vi "Read InTemperatureRange.vi"(8 "error in (no error)":errorcluster, 11 "CoolerControler in":refnum<class "CoolerControler.lvclass">) -> (0 "error out":errorcluster, 2 "InTemperatureRange":dbl=3.0, 3 "CoolerControler out":refnum<class "CoolerControler.lvclass">)   [LabVIEW 2016, in "CoolerControler.lvclass"]
uses:
  CoolerControler.lvclass
  CoolerControler.lvclass/CoolerControler.ctl
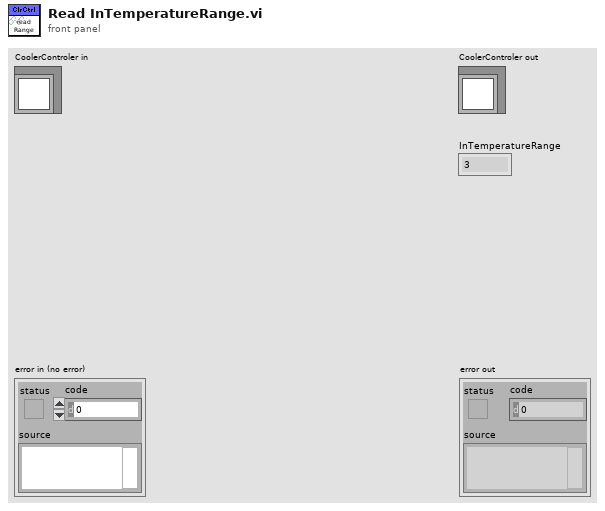
[diagram p1: front panel]
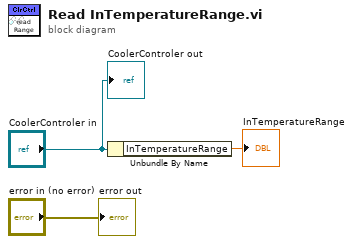
[diagram p0: block diagram]
diagram:
  n1 = Unbundle By Name("CoolerControler in") -> ("InTemperatureRange"=→"InTemperatureRange":dbl)
  "error out" <- "error in (no error)"
  "CoolerControler out" <- "CoolerControler in"
